vi "Update Status with Error Info.vi"(8 "error in (no error)":errorcluster, 11 "LabVIEW Build Script":refnum<class "LabVIEW Build Script.lvclass">) -> (3 "Error":bool)   [LabVIEW 2021, in "LabVIEW Build Script.lvclass"]
uses:
  LabVIEW Build Script.lvclass
  LabVIEW Build Script.lvclass/LabVIEW Build Script.ctl
  <vilib>/CIF Foundation/CIF Utilities/Errors/Errors_CIF_U.lvlib
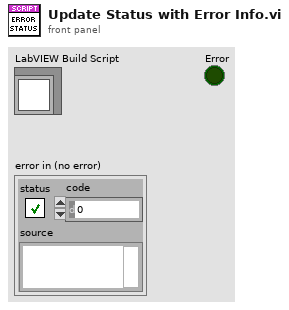
[diagram p1: front panel]
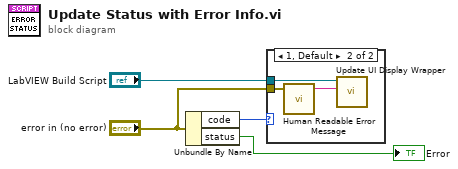
[diagram p0: block diagram]
diagram:
  n1 = Unbundle By Name("error in (no error)") -> ("code"=w4:i32, "status"=→"Error":bool)
  n2 = case shown="1, Default" w4 {
    tunnel: "error in (no error)" -> [_ w7]
    tunnel: "LabVIEW Build Script" -> [_ w5]
    frame 0 {
    }
    frame 1, Default {
      n3 = call <vilib>:"Human Readable Error Message.vi"("error in (no error)"=w7) -> ("Human readable error message"=w6:string)  [unwired: 4 in]
      n4 = call "Update UI Display Wrapper.vi"("Update for Display"=w6, "LabVIEW Build Script in"=w5) -> ()  [unwired: 9 in, 1 out]
    }
  }
